vi "布尔字符串转换.vi"(0 "布尔":bool, 5 "布尔 2":bool, 7 "布尔 3":bool, 9 "布尔 4":bool, 11 "布尔 5":bool) -> (4 "连接的字符串":string)   [LabVIEW 2017]
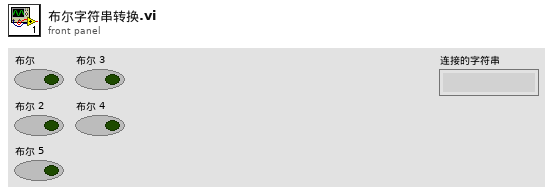
[diagram p1: front panel]
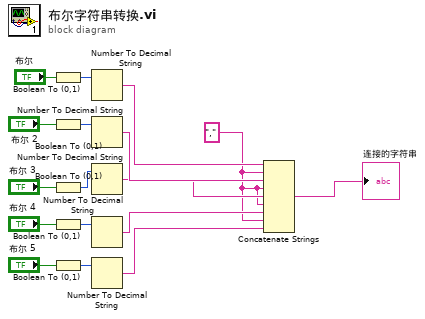
[diagram p0: block diagram]
diagram:
  w1 = "," ("字符串")
  n1 = Boolean To (0,1)(Boolean="布尔") -> (0, 1=w17:i16)
  n2 = Boolean To (0,1)(Boolean="布尔 2") -> (0, 1=w16:i16)
  n3 = Boolean To (0,1)(Boolean="布尔 3") -> (0, 1=w2:i16)
  n4 = Boolean To (0,1)(Boolean="布尔 4") -> (0, 1=w15:i16)
  n5 = Boolean To (0,1)(Boolean="布尔 5") -> (0, 1=w9:i16)
  n6 = Number To Decimal String(number=w17) -> (decimal integer string=w8:string)  [unwired: 1 in]
  n7 = Number To Decimal String(number=w16) -> (decimal integer string=w7:string)  [unwired: 1 in]
  n8 = Number To Decimal String(number=w2) -> (decimal integer string=w6:string)  [unwired: 1 in]
  n9 = Number To Decimal String(number=w15) -> (decimal integer string=w5:string)  [unwired: 1 in]
  n10 = Number To Decimal String(number=w9) -> (decimal integer string=w4:string)  [unwired: 1 in]
  n11 = Concatenate Strings(w8, w1, w7, w1, w6, w1, w5, w1, w4) -> (→"连接的字符串":string)
